vi "Test Timer.vi"() -> ()   [LabVIEW 2020]
uses:
  Time/Timer/Method/New.vi
  Time/Timer/Method/Reset.vi
  Time/Timer/Method/Wait.vi
  Time/Timer/Method/Pause.vi
  Time/Timer/Method/Continue.vi
  Time/Timer/Method/Delete.vi
  Time/Timer/Timer.lvclass
panel:
  in  "continue":bool
  in  "pause":bool
  out "elapsed time(s)":dbl
  in  "error in (no error)":errorcluster
  out "error out":errorcluster
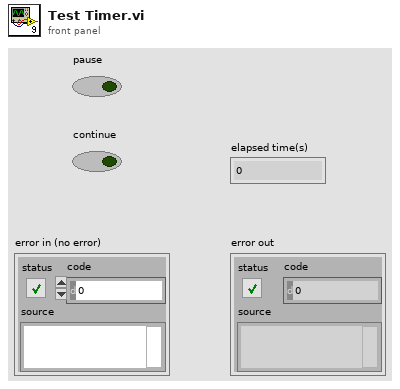
[diagram p1: front panel]
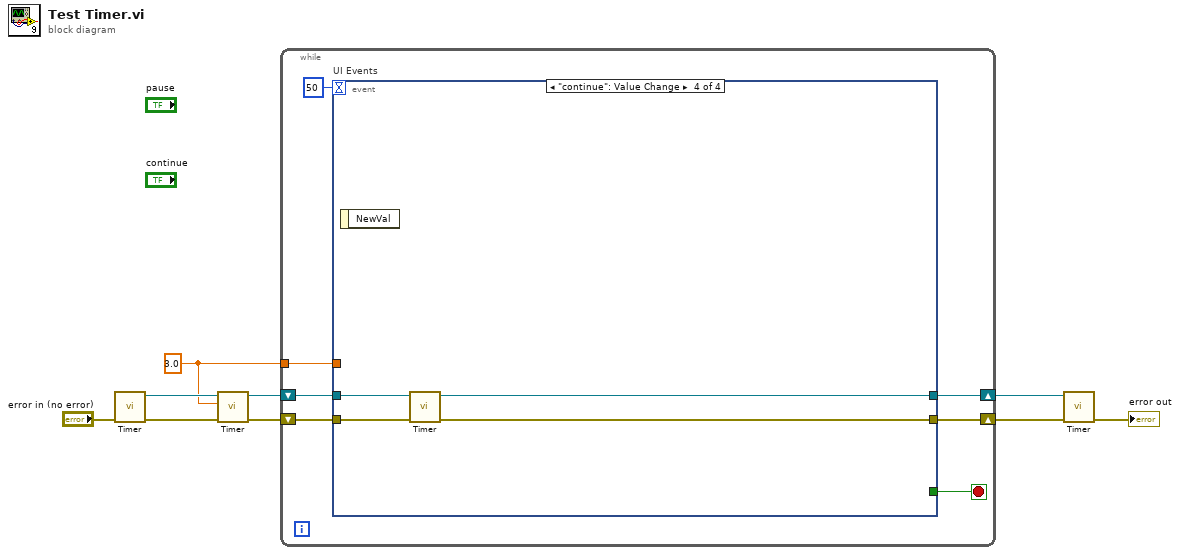
[diagram p0: block diagram]
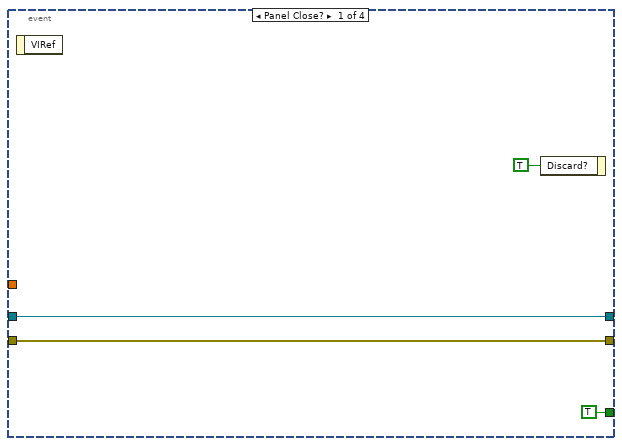
[diagram p2: hidden frame]
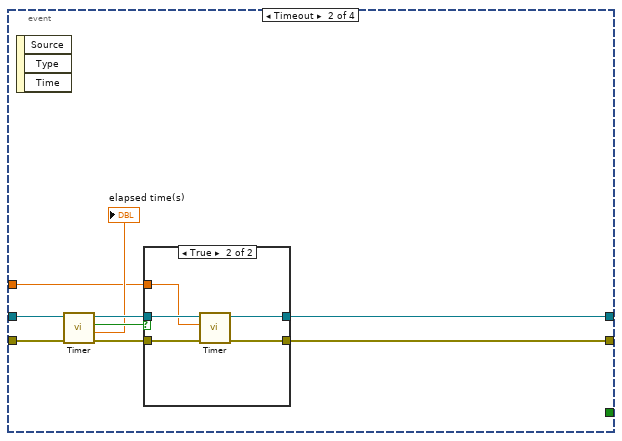
[diagram p3: hidden frame]
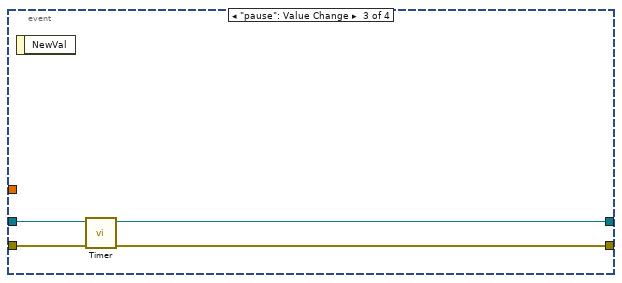
[diagram p5: hidden frame]
diagram:
  w1 = 3.0 ("target time(s)")
  n1 = call-poly "Timer.vi"("error in (no error)"="error in (no error)") -> ("error out"=w5:errorcluster, "Timer out"=w4:refnum<class "Timer.lvclass">)  [unwired: 9 in]
  n2 = call-poly "Timer.vi"("error in (no error)"=w5, "target time(s)"=w1, "Timer in"=w4) -> ("error out"=w2:errorcluster, "Timer out"=w3:refnum<class "Timer.lvclass">)  [unwired: 7 in]
  n3 = while {
    shift-right: [w14] -> w8
    shift-left: w2 -> [w15]
    shift-right: [w12] -> w6
    shift-left: w3 -> [w13]
    tunnel: w1 -> [w11]
    stop <- w16 stop-if-true
    n4 = event "UI Events" shown="[3] \"continue\": Value Change" {
      selector: _ -> [_ _ _ _]
      dyn-events: _ -> [_ _ _ _]
      timeout: 50 -> [_ _ _ _]
      tunnel: [TRUE ("stop") _ _ _] -> w16
      tunnel: w15 -> [w19 w29 w40 w44]
      tunnel: [w19 w21 w37 w41] -> w14
      tunnel: w13 -> [w17 w28 w39 w43]
      tunnel: [w17 w22 w38 w42] -> w12
      tunnel: w11 -> [_ w23 _ _]
      event Panel Close? {
        n5 = event-data() -> ()  [unwired: 1 in, 1 out]
        n6 = event-data("Discard?"=TRUE) -> ()  [unwired: 1 in, 1 out]
      }
      event Timeout {
        n7 = event-data() -> ()  [unwired: 1 in, 3 out]
        n8 = call-poly "Timer.vi"("error in (no error)"=w29, "Timer in"=w28) -> ("error out"=w24:errorcluster, "elapsed time(s)"=→"elapsed time(s)":dbl, "timeout"=w26:bool, "Timer out"=w27:refnum<class "Timer.lvclass">)  [unwired: 6 in]
        n9 = case shown="True" w26 {
          tunnel: w27 -> [w31 w35]
          tunnel: w24 -> [w30 w36]
          tunnel: w23 -> [_ w34]
          tunnel: [w31 w33] -> w22
          tunnel: [w30 w32] -> w21
          frame False {
          }
          frame True {
            n10 = call-poly "Timer.vi"("error in (no error)"=w36, "target time(s)"=w34, "Timer in"=w35) -> ("error out"=w32:errorcluster, "Timer out"=w33:refnum<class "Timer.lvclass">)  [unwired: 7 in]
          }
        }
      }
      event "pause": Value Change {
        n11 = event-data() -> ()  [unwired: 1 in, 1 out]
        n12 = call-poly "Timer.vi"("error in (no error)"=w40, "Timer in"=w39) -> ("error out"=w37:errorcluster, "Timer out"=w38:refnum<class "Timer.lvclass">)  [unwired: 8 in]
      }
      event "continue": Value Change {
        n13 = event-data() -> ()  [unwired: 1 in, 1 out]
        n14 = call-poly "Timer.vi"("error in (no error)"=w44, "Timer in"=w43) -> ("error out"=w41:errorcluster, "Timer out"=w42:refnum<class "Timer.lvclass">)  [unwired: 8 in]
      }
    }
  }
  n15 = call-poly "Timer.vi"("error in (no error)"=w8, "Timer in"=w6) -> ("error out"=→"error out":errorcluster)  [unwired: 9 in]
